vi "MGCC_LoadFcst.vi"(1 "InputTimeSeries":dbl[][](array[numeric])) -> (0 "OutputTimeSeries":dbl[][](array[numeric]))   [LabVIEW 2016]
doc: "This VI realizes the load forecasting function in the MGCC. Input is a historical time series of load data in 15 min intervals. Output is 96-point-ahead (24 hrs) of the load. This VI uses a simple AR model for forecasting."
uses:
  <vilib>/addons/Time Series Analysis/Modeling and Prediction.llb/TSA AR Modeling Order (Array).vi
  <vilib>/addons/Time Series Analysis/Modeling and Prediction.llb/TSA ARMA Modeling (Array).vi
  <vilib>/addons/Time Series Analysis/Modeling and Prediction.llb/TSA ARMA Prediction (Array).vi
  <vilib>/addons/_Advanced Signal Processing/NI_AdvSigProcTSA.lvlib
panel:
  out "standard deviation":dbl[][](array[numeric]) format="%.4f"
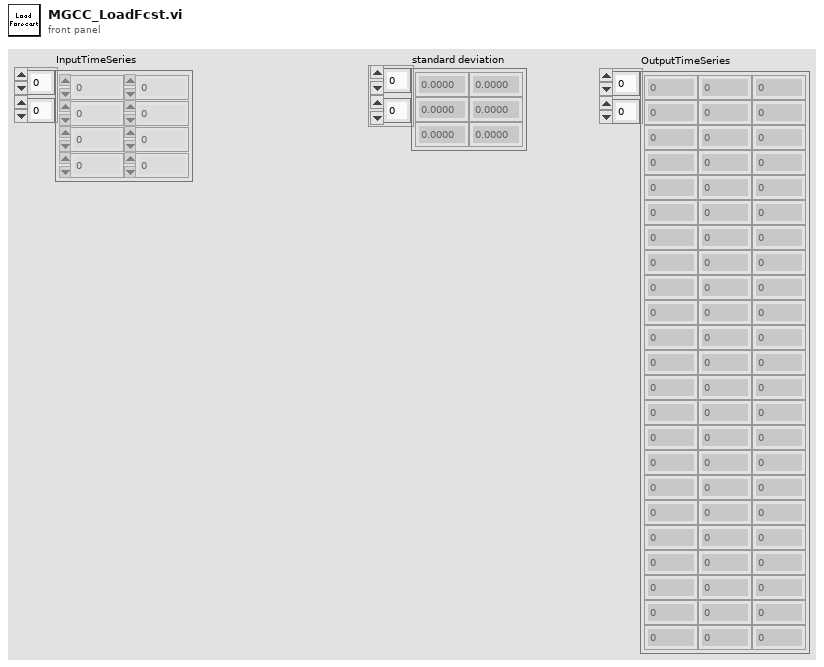
[diagram p1: front panel]
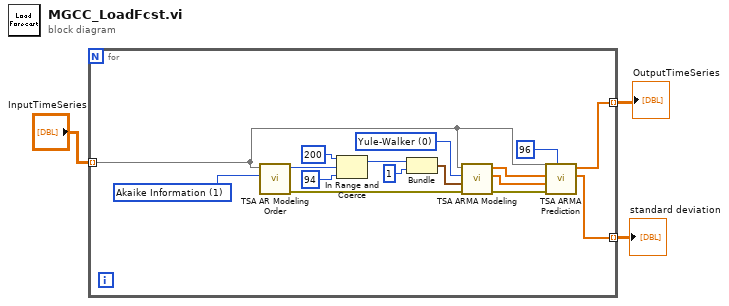
[diagram p0: block diagram]
diagram:
  n1 = for {
    tunnel: "InputTimeSeries" -> [w4] mode=indexing
    tunnel: [w6] -> w2 mode=indexing
    tunnel: [w5] -> w1 mode=indexing
    w14 = 1 items=["Final Prediction Error"=0, "Akaike Information"=1, "Bayesian Information"=4, "Minimal Description Length"=2, "Phi Criterion"=3, "-"=-1, "Partial Correlation Function"=6] ("method")
    w15 = u16 0 items=["Yule-Walker", "High order AR", "Polynomial"] ("method")
    n2 = call-poly <vilib>:"TSA AR Modeling Order.vi"("method"=w14, "Xt"=w4) -> ("error out"=w13:errorcluster, "optimal AR order"=w10:i32)  [unwired: 7 in, 1 out]
    n3 = In Range and Coerce(upper limit=200, x=w10, lower limit=94) -> (coerced(x)=w7:i32)  [unwired: 1 out]
    n4 = Bundle("upper limit"=w7, 1) -> (w11:cluster{"upper limit":i32, i32})  [unwired: 1 in]
    n5 = call-poly <vilib>:"TSA ARMA Modeling.vi"("error in (no error)"=w13, "ARMA order"=w11, "method"=w15, "Xt"=w4) -> ("error out"=w18:errorcluster, "MA coefficients"=w16:dbl[], "AR coefficients"=w17:dbl[])  [unwired: 4 in, 1 out]
    n6 = call-poly <vilib>:"TSA ARMA Prediction.vi"("number of points"=96, "error in (no error)"=w18, "MA coefficients"=w16, "AR coefficients"=w17, "Xt"=w4) -> ("standard deviation"=w5:dbl[], "predicted series"=w6:dbl[])  [unwired: 4 in, 1 out]
  }
  "OutputTimeSeries" <- w2
  "standard deviation" <- w1
